vi "Color Sensor V3 Get Color.vi"(8 "error in (no error)":errorcluster, 11 "ColorSensorDevRef":T1={"I2CDevRef"={"DevStatus"={"status"=FALSE, "code"=0, "source"=""}, "Device Address"=0, "Handle"=0, "I2C Bus"=enum."Invalid"}} {"I2CDevRef"."Device Address" format="%.0x"}) -> (0 "error out":errorcluster, 1 "Normalized Color":cluster{"R":dbl, "G":dbl, "B":dbl}, 2 "Color":u32(colorbox), 3 "ColorSensorDevRef out":T1={"I2CDevRef"={"DevStatus"={"status"=FALSE, "code"=0, "source"=""}, "Device Address"=0, "Handle"=0, "I2C Bus"=enum."Invalid"}} {"I2CDevRef"."Device Address" format="%.0x"})   [LabVIEW 2023]
uses:
  Typedef/Color Sensor V3 DevRef.ctl
  <vilib>/Rock Robotics/WPI/I2C/WPI_I2CDevRef.ctl
  <vilib>/Rock Robotics/SystemInterfaces/i2clib/i2c_bus.ctl
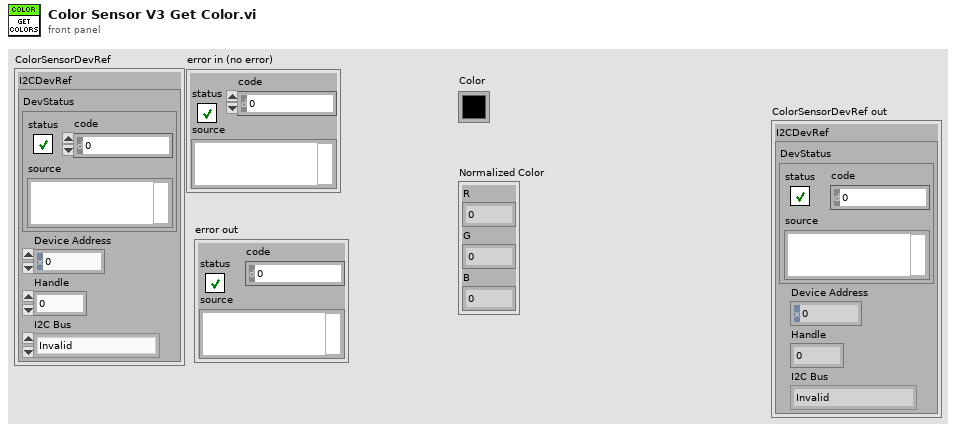
[diagram p1: front panel]
types:
  T1 = typedef "Color Sensor V3 DevRef.ctl" = cluster{"I2CDevRef":T2}
  T2 = typedef "WPI_I2CDevRef.ctl" = cluster{"DevStatus":errorcluster, "Device Address":u8, "Handle":i32, "I2C Bus":T3}
  T3 = typedef "i2c_bus.ctl" = enum16{"I2C On-Board", "I2C MXP", "Invalid"}
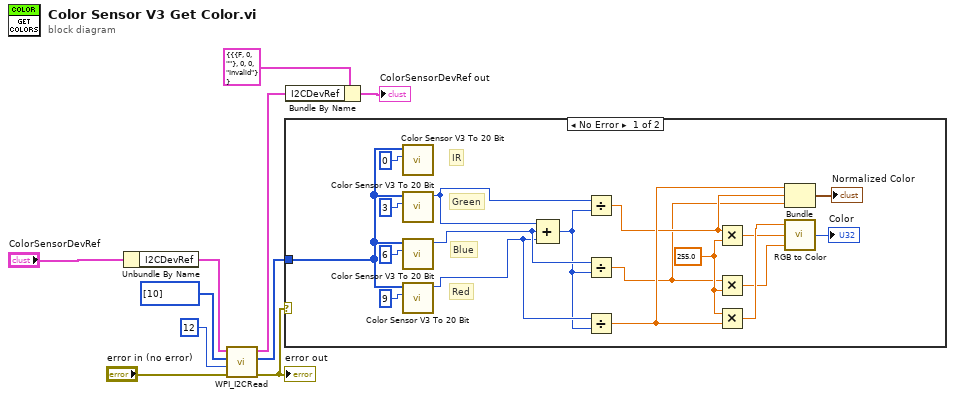
[diagram p0: block diagram]
diagram:
  n1 = Unbundle By Name("ColorSensorDevRef") -> ("I2CDevRef"=w7:T2)
  n2 = call <vilib>:"WPI_I2CRead.vi"("error in (no error)"="error in (no error)", "I2CBytesToRead"=u8 12, "I2CRegister"=u8[] [10], "I2CDevRef"=w7) -> ("error out"=w5:errorcluster, "Data Out"=w4:u8[], "I2CDevRef"=w2:T2)  [unwired: 5 in]
  "error out" <- w5
  n3 = case shown="No Error" w5 {
    tunnel: w4 -> [w28 _]
    frame No Error {
      w18 = 255.0 ("y")
      # "Red"
      # "Blue"
      # "Green"
      # "IR"
      n4 = call "Color Sensor V3 To 20 Bit.vi"("index (0)"=0 ("index"), "array"=w28) -> ()  [unwired: 9 in, 1 out]
      n5 = call "Color Sensor V3 To 20 Bit.vi"("index (0)"=3 ("index"), "array"=w28) -> ("Result"=w23:u32)  [unwired: 9 in]
      n6 = call "Color Sensor V3 To 20 Bit.vi"("index (0)"=6 ("index"), "array"=w28) -> ("Result"=w22:u32)  [unwired: 9 in]
      n7 = call "Color Sensor V3 To 20 Bit.vi"("index (0)"=9 ("index"), "array"=w28) -> ("Result"=w21:u32)  [unwired: 9 in]
      n8 = Compound Arithmetic op=ADD(w23, w22, w21) -> (w20:u32)
      n9 = Divide(x=w23, y=w20) -> (x/y=w12:dbl)
      n10 = Divide(x=w22, y=w20) -> (x/y=w11:dbl)
      n11 = Divide(x=w21, y=w20) -> (x/y=w13:dbl)
      n12 = Multiply(x=w12, y=w18) -> (x*y=w16:dbl)
      n13 = Multiply(x=w11, y=w18) -> (x*y=w15:dbl)
      n14 = Multiply(x=w18, y=w13) -> (x*y=w17:dbl)
      n15 = Bundle(w13, w12, w11) -> (→"Normalized Color":cluster{dbl, dbl, dbl})  [unwired: 1 in]
      n16 = call <vilib>:"RGB to Color.vi"("B"=w15, "G"=w16, "R"=w17) -> ("Color"=→"Color":u32)
    }
    frame Error {
    }
  }
  n17 = Bundle By Name(cluster=T1 {"I2CDevRef"={"DevStatus"={"status"=FALSE, "code"=0, "source"=""}, "Device Address"=0, "Handle"=0, "I2C Bus"=enum."Invalid"}} ("ColorSensorDevRef 2"), "I2CDevRef"=w2) -> (→"ColorSensorDevRef out":T1)
